vi "Read Configure Tester.vi"(8 "error in":errorcluster, 11 "Potting Procedure in":refnum<class "Potting Procedure.lvclass">) -> (0 "error out":errorcluster, 2 "Configure Tester":T1, 3 "Potting Procedure out":refnum<class "Potting Procedure.lvclass">)   [LabVIEW 2011, in "Potting Procedure.lvclass"]
uses:
  Potting Procedure.lvclass
  Type Definitions/Configure Tester.ctl
  UI typedefs/Chuck Control.ctl
  UI typedefs/Chuck Slot Control.ctl
  Potting Procedure.lvclass/Potting Procedure.ctl
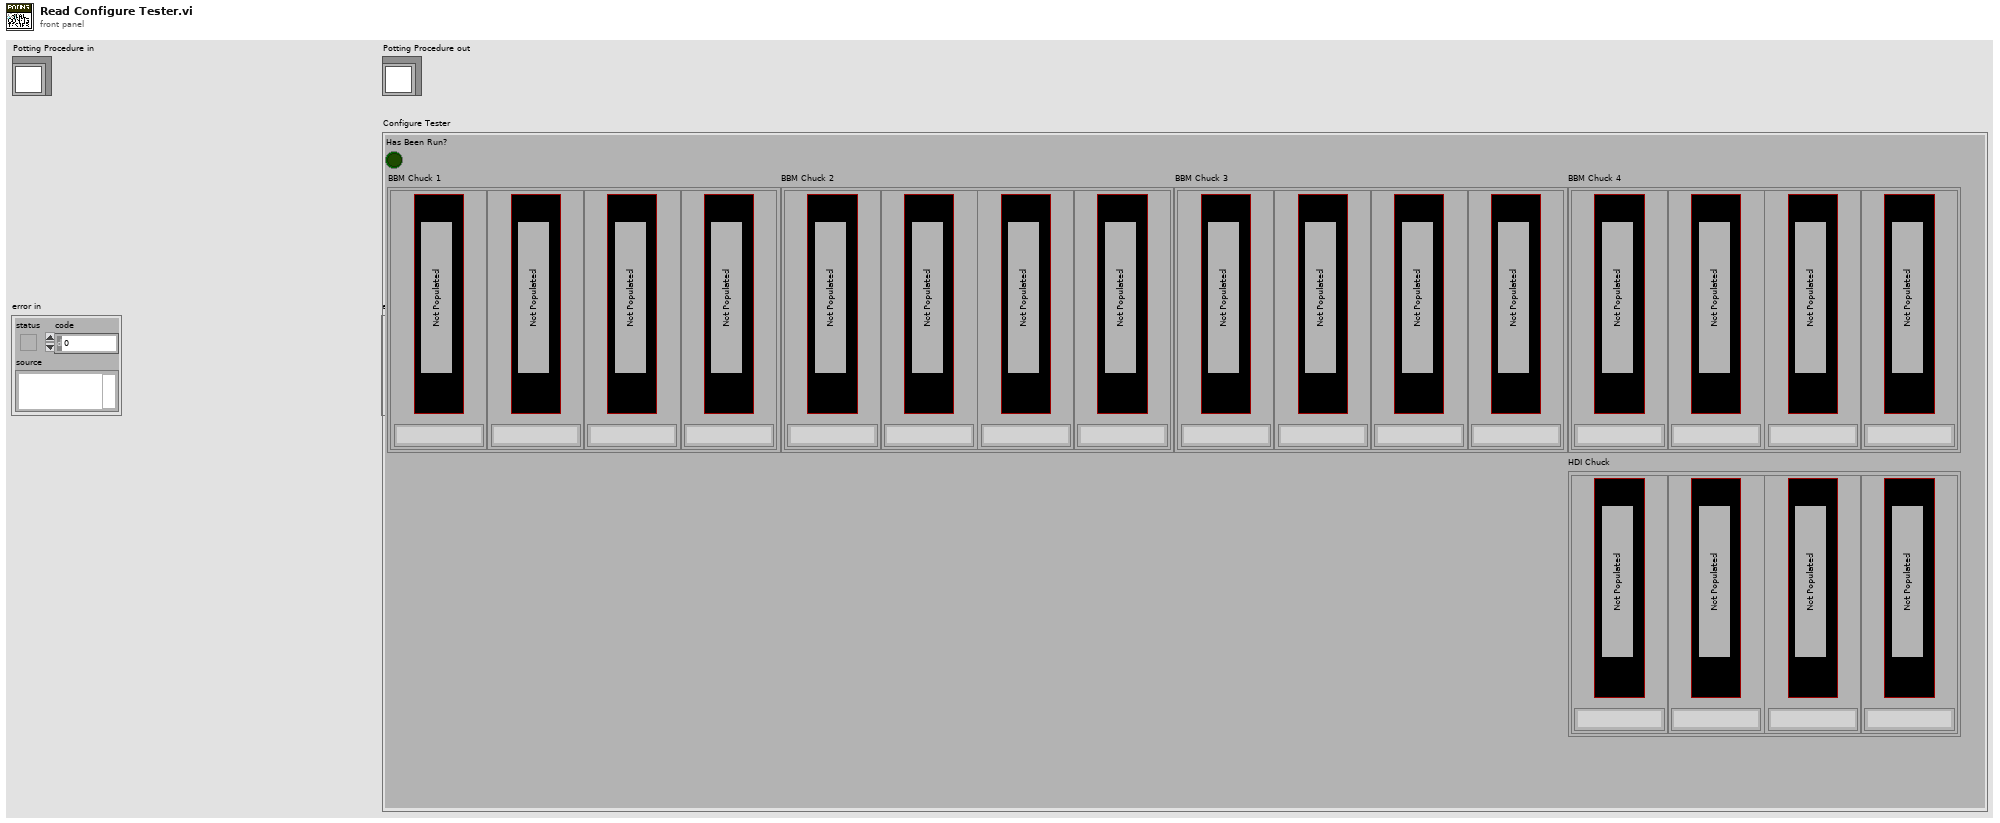
[diagram p1: front panel]
types:
  T1 = typedef "Configure Tester.ctl" = cluster{"Has Been Run?":bool, "BBM Chuck 1":T2, "BBM Chuck 2":T2, "BBM Chuck 3":T2, "BBM Chuck 4":T2, "HDI Chuck":T2}
  T2 = typedef "Chuck Control.ctl" = cluster{"Slot 1":T3, "Slot 2":T3, "Slot 3":T3, "Slot 4":T3}
  T3 = typedef "Chuck Slot Control.ctl" = cluster{"Slot Populated":bool, "S/N":string}
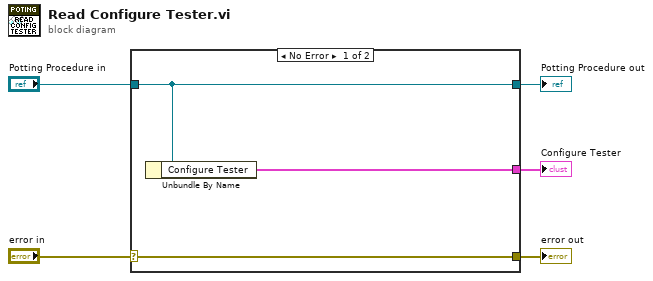
[diagram p0: block diagram]
diagram:
  n1 = case shown="No Error" "error in" {
    selector: "error in" -> [w8 w9]
    tunnel: [w8 w9] -> w4
    tunnel: [w7 w10] -> w2
    tunnel: "Potting Procedure in" -> [w7 w10]
    tunnel: [w6 _] -> w1
    frame No Error {
      n2 = Unbundle By Name(w7) -> ("Configure Tester"=w6:T1)
    }
    frame Error {
    }
  }
  "error out" <- w4
  "Potting Procedure out" <- w2
  "Configure Tester" <- w1
